vi "Settings To JSON.vi"(8 "error in":errorcluster, 9 "Items (DO NOT CONNECT)":string[](array[string]), 10 "Path":path, 11 "Object":variant) -> (0 "error out":errorcluster, 2 "JSON string":string, 3 "Items Out":string[](array[string]))   [LabVIEW 2023, in "Abstract Hardware.lvlib" / "Base Hardware.lvclass"]
uses:
  Base Hardware.lvclass
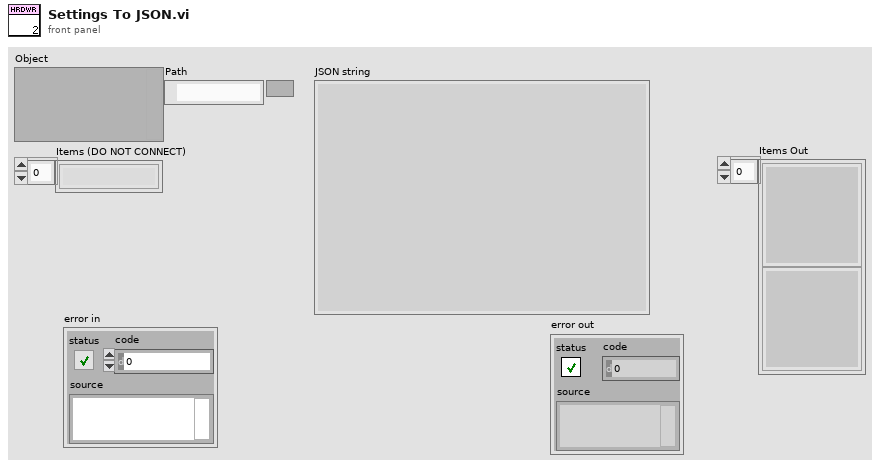
[diagram p1: front panel]
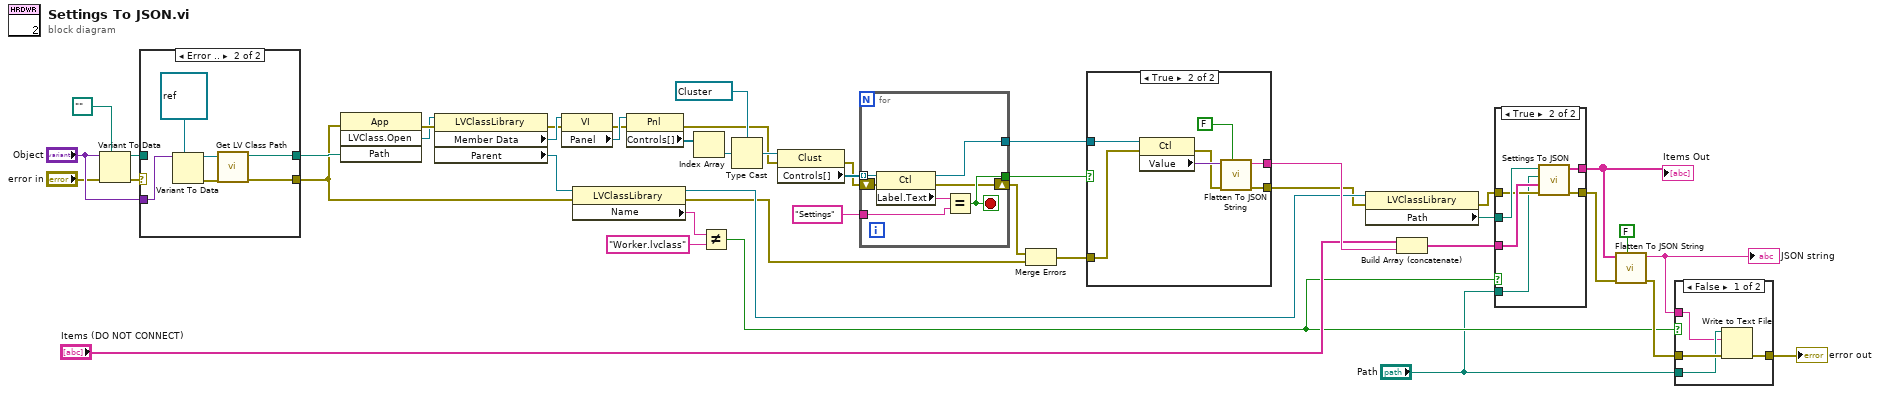
[diagram p0: block diagram]
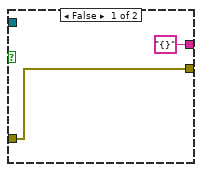
[diagram p5: hidden frame]
diagram:
  n1 = Variant To Data(error in="error in", type=path "", Variant="Object") -> (data=w26:path, error out=w28:errorcluster)
  n2 = case shown="Error .." w28 {
    selector: w28 -> [w45 _]
    tunnel: [w46 w48] -> w27
    tunnel: w26 -> [w46 _]
    tunnel: "Object" -> [_ w51]
    tunnel: [w45 w47] -> w14
    frame No Error {
    }
    frame Error {
      n3 = Variant To Data(type=refnum<class> refnum ("LabVIEW Object"), Variant=w51) -> (data=w49:refnum<class>, error out=w52:errorcluster)  [unwired: 1 in]
      n4 = call <vilib>:"Get LV Class Path.vi"("error in (no error)"=w52, "object"=w49) -> ("error out"=w47:errorcluster, "class path"=w48:path)  [unwired: 8 in]
    }
  }
  n5 = invoke class="App" method="LVClass.Open"(error in=w14, "Path"=w27) -> (error out=w18:errorcluster, "LVClass.Open"=w17:refnum<vi>)  [unwired: 2 in, 2 out]
  n6 = property class="LVClassLibrary"(reference=w17, error in=w18) -> (error out=w37:errorcluster, "Member Data"=w38:refnum<vi>, "Parent"=w35:refnum<vi>)  [unwired: 1 out]
  n7 = property class="VI"(reference=w38, error in=w37) -> (error out=w36:errorcluster, "Panel"=w44:refnum<vi>)  [unwired: 1 out]
  n8 = property class="LVClassLibrary"(reference=w35, error in=w14) -> (reference out=w23:refnum<vi>, error out=w12:errorcluster, "Name"=w33:string)
  n9 = property class="Pnl"(reference=w44, error in=w36) -> (error out=w16:errorcluster, "Controls[]"=w43:refnum<vi>[])  [unwired: 1 out]
  n10 = Index Array(array=w43) -> (element=w42:refnum<vi>)  [unwired: 1 in]
  n11 = Not Equal?(x=w33, y="Worker.lvclass") -> (x != y?=w4:bool)
  n12 = Type Cast(type=refnum<vi> refnum ("reference"), x=w42) -> (*(type *) &x=w40:refnum<vi>)
  n13 = property class="Clust"(reference=w40, error in=w16) -> (error out=w15:errorcluster, "Controls[]"=w39:refnum<vi>[])  [unwired: 1 out]
  n14 = for {
    tunnel: w39 -> [w59] mode=indexing
    tunnel: "Settings" -> [w57]
    tunnel: [w56] -> w30
    tunnel: [w55] -> w31
    shift-right: [w53] -> w13
    shift-left: w15 -> [w54]
    stop <- w55 stop-if-true
    n15 = property class="Ctl"(reference=w59, error in=w54) -> (reference out=w56:refnum<vi>, error out=w53:errorcluster, "Label.Text"=w58:string)
    n16 = Equal?(x=w58, y=w57) -> (x = y?=w55:bool)
  }
  n17 = Merge Errors(w13, w12) -> (w11:errorcluster)
  n18 = case shown="True" w31 {
    tunnel: w30 -> [_ w68]
    tunnel: ["{}" ("JSON String") w66] -> w24
    tunnel: w11 -> [w60 w65]
    tunnel: [w60 w63] -> w10
    frame False {
    }
    frame True {
      n19 = property class="Ctl"(reference=w68, error in=w65) -> (error out=w62:errorcluster, "Value"=w67:variant)  [unwired: 1 out]
      n20 = call <vilib>:"Flatten To JSON String.vi"("Multiline (T)"=FALSE, "error in"=w62, "Variant"=w67) -> ("error out"=w63:errorcluster, "JSON String"=w66:string)  [unwired: 7 in]
    }
  }
  n21 = property class="LVClassLibrary"(reference=w23, error in=w10) -> (error out=w7:errorcluster, "Path"=w21:path)  [unwired: 1 out]
  n22 = Build Array (concatenate)("Items (DO NOT CONNECT)", w24) -> (w20:string[])
  n23 = case shown="True" w4 {
    tunnel: w21 -> [_ w76]
    tunnel: w20 -> [w70 w74]
    tunnel: [w70 w75] -> w19
    tunnel: w7 -> [w69 w73]
    tunnel: [w69 w72] -> w6
    tunnel: "Path" -> [_ w71]
    frame False {
    }
    frame True {
      n24 = call "Settings To JSON.vi"("error in"=w73, "Items (DO NOT CONNECT)"=w74, "Path"=w71, "Object"=w76) -> ("error out"=w72:errorcluster, "Items Out"=w75:string[])  [unwired: 5 in, 1 out]
    }
  }
  "Items Out" <- w19
  n25 = call <vilib>:"Flatten To JSON String.vi"("Multiline (T)"=FALSE, "error in"=w6, "Variant"=w19) -> ("error out"=w5:errorcluster, "JSON String"=w3:string)  [unwired: 7 in]
  "JSON string" <- w3
  n26 = case shown="False" w4 {
    tunnel: w5 -> [w80 w81]
    tunnel: w3 -> [w78 _]
    tunnel: "Path" -> [w79 _]
    tunnel: [w77 w81] -> w2
    frame False {
      n27 = Write to Text File(file (use dialog)=w79, text=w78, error in=w80) -> (error out=w77:errorcluster)  [unwired: 1 in, 2 out]
    }
    frame True {
    }
  }
  "error out" <- w2
